vi "EXAMPLE_PARSEFILE.vi"() -> ()   [LabVIEW 2017]
uses:
  src/TagDB/_Support/Disk/tagdbfile-v3.1.ctl
  src/TagDB/TagDB.lvlib
panel:
  out "version":string
  in  "Listbox":i32(listbox)
  out "Variant":variant
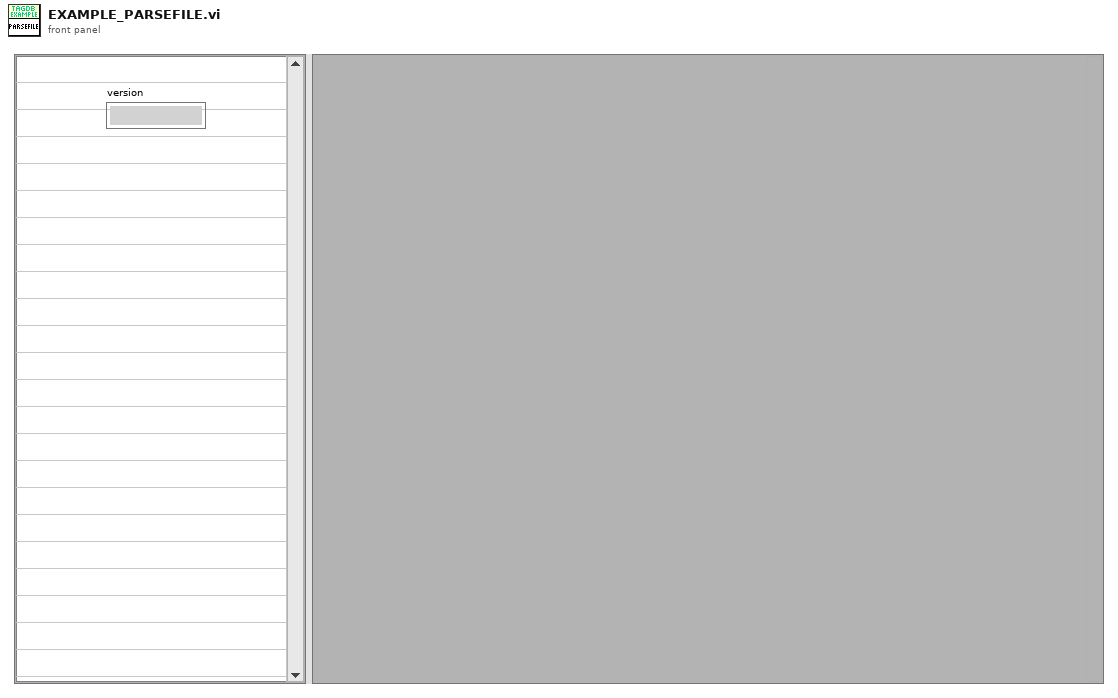
[diagram p1: front panel]
types:
  T1 = typedef "TagDB.lvlib/tagdbfile-v3.1.ctl" = cluster{"version":string, "db":variant[]}
  T2 = enum16{"open", "replace", "create", "open or create", "replace or create", "replace or create with confirmation"}
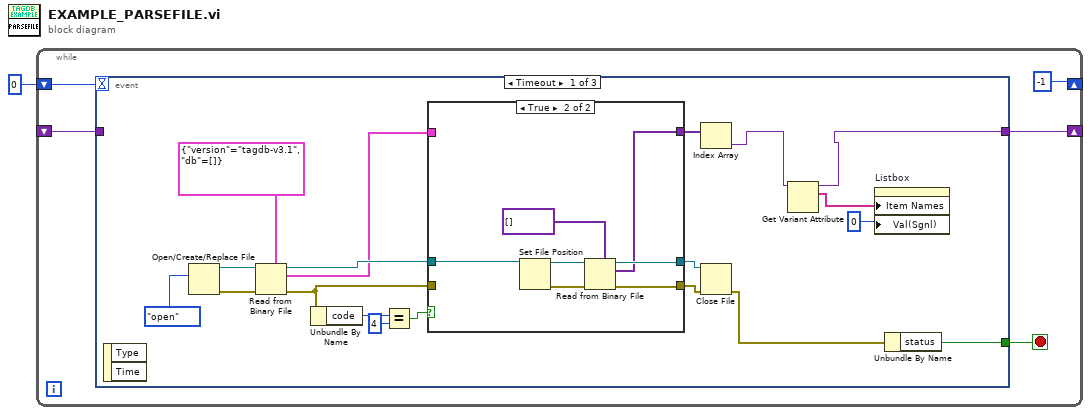
[diagram p0: block diagram]
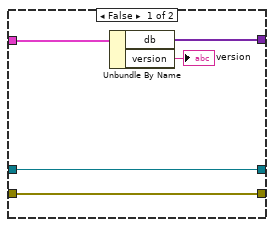
[diagram p2: hidden frame]
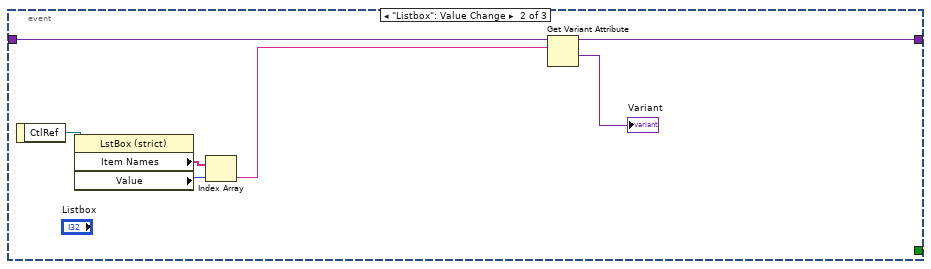
[diagram p3: hidden frame]
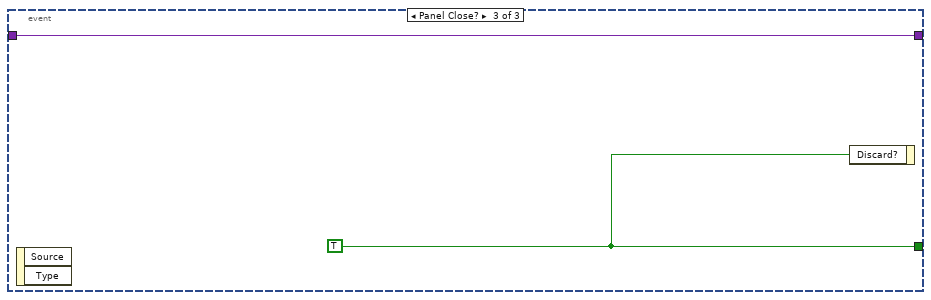
[diagram p4: hidden frame]
diagram:
  n1 = while {
    shift-right: [-1] -> _
    shift-left: 0 -> [w5]
    shift-right: [w3] -> _
    shift-left: _ -> [w2]
    stop <- w6 stop-if-true
    n2 = event shown="[0] Timeout" {
      selector: _ -> [_ _ _]
      dyn-events: _ -> [_ _ _]
      timeout: w5 -> [_ _ _]
      tunnel: [w24 _ w46] -> w6
      tunnel: [w7 w39 w45] -> w3
      tunnel: w2 -> [_ w41 w45]
      event Timeout {
        n3 = event-data() -> ()  [unwired: 1 in, 2 out]
        n4 = Open/Create/Replace File(operation (0:open)=T2."open") -> (refnum out=w23:refnum<file>, error out=w22:errorcluster)  [unwired: 5 in, 1 out]
        n5 = Read from Binary File(5:T1 {"version"="tagdb-v3.1", "db"=[]} ("tagdb-file-v3.1"), 8:w22, 11:w23) -> (0:w15:errorcluster, 2:w17:T1, 3:w19:refnum<file>)  [unwired: 3 in, 1 out]
        n6 = Unbundle By Name(w15) -> ("code"=w14:i32)
        n7 = Equal?(x=w14, y=4) -> (x = y?=w12:bool)
        n8 = case shown="True" w12 {
          tunnel: [w30 w33] -> w20
          tunnel: w19 -> [w30 w37]
          tunnel: [w29 w34] -> w18
          tunnel: [w28 w31] -> w10
          tunnel: w17 -> [w27 _]
          tunnel: w15 -> [w29 _]
          frame False {
            n9 = Unbundle By Name(w27) -> ("db"=w28:variant[], "version"=→"version":string)
          }
          frame True {
            n10 = Set File Position(refnum=w37) -> (refnum out=w35:refnum<file>, error out=w36:errorcluster)  [unwired: 3 in]
            n11 = Read from Binary File(5:variant[] [] ("Array"), 8:w36, 11:w35) -> (0:w34:errorcluster, 2:w31:variant[], 3:w33:refnum<file>)  [unwired: 3 in, 1 out]
          }
        }
        n12 = Index Array(array=w10) -> (element=w8:variant)  [unwired: 1 in]
        n13 = Close File(refnum=w20, error in=w18) -> (error out=w11:errorcluster)  [unwired: 1 out]
        n14 = Get Variant Attribute(Variant=w8) -> (duplicate Variant=w7:variant, names=w9:string[])  [unwired: 3 in, 2 out]
        n15 = property on="Listbox" class="LstBox (strict)"("Item Names"=w9, "Val(Sgnl)"=0 ("Value (Signaling)")) -> ()  [unwired: 2 in, 2 out]
        n16 = Unbundle By Name(w11) -> ("status"=w24:bool)
      }
      event "Listbox": Value Change {
        n17 = event-data() -> ("CtlRef"=w44:refnum<vi>)  [unwired: 1 in]
        n18 = property class="LstBox (strict)"(reference=w44) -> ("Item Names"=w42:string[], "Value"=w43:i32)  [unwired: 1 in, 2 out]
        n19 = Index Array(array=w42, index=w43) -> (element=w40:string)
        n20 = Get Variant Attribute(Variant=w41, name=w40) -> (duplicate Variant=w39:variant, value=→"Variant":variant)  [unwired: 2 in, 2 out]
      }
      event Panel Close? {
        w46 = TRUE
        n21 = event-data() -> ()  [unwired: 1 in, 2 out]
        n22 = event-data("Discard?"=w46) -> ()  [unwired: 1 in, 1 out]
      }
    }
  }
